vi "Msg.vi"(7 "Actor in":refnum<class "Actor.lvclass">, 11 "Actor Create Msg Strategy in":refnum<class "Actor Create Msg Strategy.lvclass">) -> (0 "error out":errorcluster, 5 "Actor out":refnum<class "Actor.lvclass">)   [LabVIEW 2021, in "Actor Create.lvlib" / "Actor Create Msg Strategy.lvclass"]
uses:
  Actor Create Msg Strategy.lvclass
  LVCAM/Actor/Actor.lvclass
  Actor Create/Actor Create.lvclass
  b9b3c3c6-ce11-415e-ad89-e7059c446d1f.vi
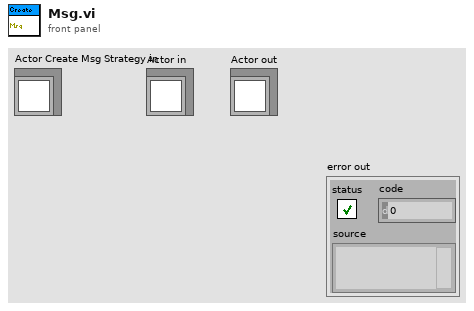
[diagram p1: front panel]
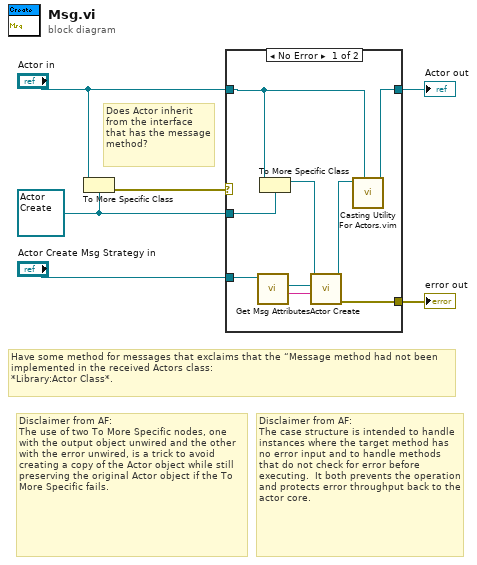
[diagram p0: block diagram]
diagram:
  w5 = refnum<class "Actor Create.lvclass"> refnum ("Create.lvlib:Create.lvclass")
  # "Does Actor inherit from the interface that has the message method?"
  # "Disclaimer from AF:\nThe use of two To More Specific nodes, one with the output object unwired and the other with the error unwired, is a trick to avoid creating a copy of the Actor object while still preserving the original Actor object if the To More Specific fails."
  # "Disclaimer from AF:\nThe case structure is intended to handle instances where the target method has no error input and to handle methods that do not check for error before executing.  It both prevents the operation and protects error throughput back to the actor core."
  # "Have some method for messages that exclaims that the “Message method had not been implemented in the received Actors class:\n*Library:Actor Class*."
  n1 = To More Specific Class(target class=w5, reference="Actor in") -> (error out=w6:errorcluster)  [unwired: 1 in, 1 out]
  n2 = case shown="No Error" w6 {
    selector: w6 -> [_ w17]
    tunnel: [w15 w17] -> w1
    tunnel: [w11 w16] -> w4
    tunnel: "Actor in" -> [w10 w16]
    tunnel: w5 -> [w13 _]
    tunnel: "Actor Create Msg Strategy in" -> [w9 _]
    frame No Error {
      n3 = call "Get Msg Attributes.vi"("Actor Create Msg Strategy in"=w9) -> ("Nested Alias"=w7:string, "Nested Actor"=w8:refnum<class "Actor.lvclass">)  [unwired: 9 in]
      n4 = To More Specific Class(target class=w13, reference=w10) -> (specific class reference=w14:refnum<class "Actor Create.lvclass">)  [unwired: 1 in, 1 out]
      n5 = call-dynamic "Actor Create.vi"("Nested Alias"=w7, "Nested Actor"=w8, "Actor Create in"=w14) -> ("error out"=w15:errorcluster, "Actor Create out"=w12:refnum<class "Actor Create.lvclass">)  [unwired: 7 in]
      n6 = call "Casting Utility For Actors.vim"("type"=w10, "Actor in"=w12) -> ("Actor out"=w11:refnum<class "Actor.lvclass">)  [unwired: 8 in, 1 out]
    }
    frame Error {
    }
  }
  "error out" <- w1
  "Actor out" <- w4
